vi "Read Collapsed_.vi"(8 "error in (no error)":errorcluster, 11 "CollapsePanel in":refnum<class "CollapsePanel.lvclass">) -> (0 "error out":errorcluster, 2 "Collapsed?":bool, 3 "CollapsePanel out":refnum<class "CollapsePanel.lvclass">)   [LabVIEW 2021, in "CollapsePanel.lvclass"]
uses:
  CollapsePanel.lvclass
  CollapsePanel.lvclass/CollapsePanel.ctl
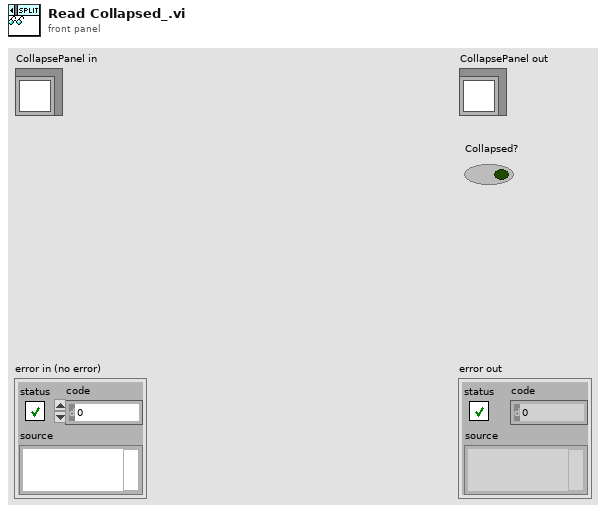
[diagram p1: front panel]
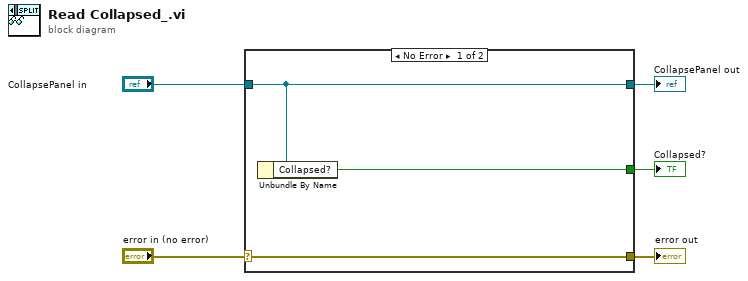
[diagram p0: block diagram]
diagram:
  n1 = case shown="No Error" "error in (no error)" {
    selector: "error in (no error)" -> [w8 w9]
    tunnel: [w8 w9] -> w4
    tunnel: [w7 w10] -> w2
    tunnel: "CollapsePanel in" -> [w7 w10]
    tunnel: [w6 _] -> w1
    frame No Error {
      n2 = Unbundle By Name(w7) -> ("Collapsed?"=w6:bool)
    }
    frame Error {
    }
  }
  "error out" <- w4
  "CollapsePanel out" <- w2
  "Collapsed?" <- w1
